vi "Matrix Inverse.vi"(11 "A":sgl[][](array[numeric])) -> (3 "Inverse A":sgl[][](array[numeric]))   [LabVIEW 2017, in "3D Plot.lvclass"]
uses:
  <vilib>/Math Plots/3D Math Plots/3D Plot/3D Plot/3D Plot.lvclass
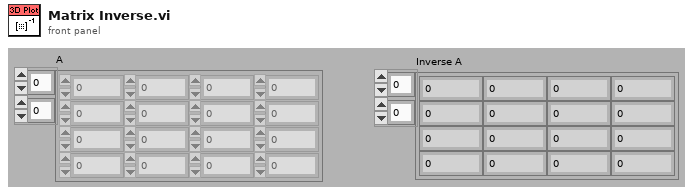
[diagram p1: front panel]
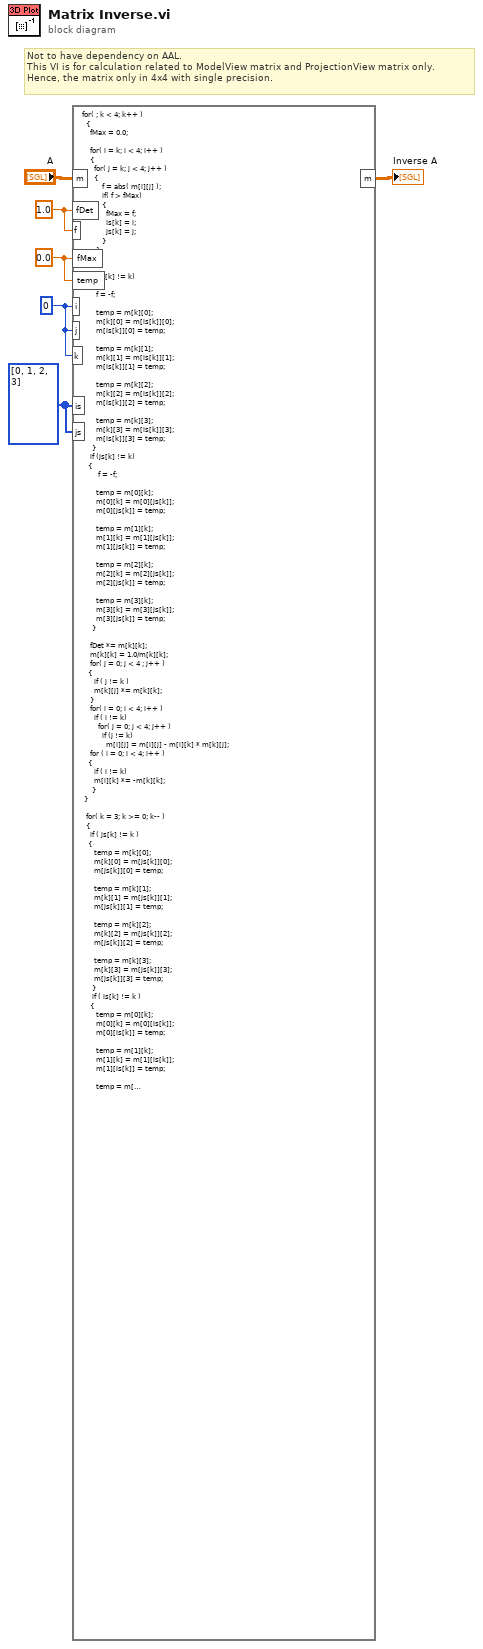
[diagram p0: block diagram]
diagram:
  w3 = 0
  w4 = i32[] [0, 1, 2, 3]
  w5 = sgl 0.0 ("input variable")
  w6 = sgl 1.0 ("input variable")
  # "Not to have dependency on AAL.\nThis VI is for calculation related to ModelView matrix and ProjectionView matrix only.\nHence, the matrix only in 4x4 with single precision."
  n1 = formula code="for( ; k < 4; k++ )\n  {\n    fMax = 0.0;\n\n    for( i = k; i < 4; i++ )\n    {\n      for( j = k; j < 4; j++ )\n      {\n          f = abs( m[i][j] );\n          if( f > fMax)\n          {\n            fMax = f;\n            is[k] = i;\n            js[k] = j;\n          }\n       }\n    }\n  \n    if (is[k] != k)\n  \t{\n       f = -f;\n\n   \t   temp = m[k][0];\n       m[k][0] = m[is[k]][0];\n       m[is[k]][0] = temp;\n\n   \t   temp = m[k][1];\n       m[k][1] = m[is[k]][1];\n       m[is[k]][1] = temp;\n\n   \t   temp = m[k][2];\n       m[k][2] = m[is[k]][2];\n       m[is[k]][2] = temp;\n\n\t      temp = m[k][3];\n       m[k][3] = m[is[k]][3];\n       m[is[k]][3] = temp; \n     }   \n    if (js[k] != k)\n  \t{\n        f = -f;\n  \n\t      temp = m[0][k];\n       m[0][k] = m[0][js[k]];\n       m[0][js[k]] = temp;\n\n\t      temp = m[1][k];\n       m[1][k] = m[1][js[k]];\n       m[1][js[k]] = temp;\n\n\t      temp = m[2][k];\n       m[2][k] = m[2][js[k]];\n       m[2][js[k]] = temp;\n\n\t      temp = m[3][k];\n       m[3][k] = m[3][js[k]];\n       m[3][js[k]] = temp;\n     }\n\n    fDet *= m[k][k];\n    m[k][k] = 1.0/m[k][k];\n    for( j = 0; j < 4 ; j++ )\n   {\n      if ( j != k )\n      m[k][j] *= m[k][k];\n    }\n    for( i = 0; i < 4; i++ )\n      if ( i != k)\n        for( j = 0; j < 4; j++ )\n          if (j != k)\n            m[i][j] = m[i][j] - m[i][k] * m[k][j];\n    for ( i = 0; i < 4; i++ )\n  \t{\n      if ( i != k)\n      m[i][k] *= -m[k][k];\n     }\n }\n\n  for( k = 3; k >= 0; k-- )\n  {\n    if ( js[k] != k )\n  \t{\n\t     temp = m[k][0];\n      m[k][0] = m[js[k]][0];\n      m[js[k]][0] = temp;\n\t  \n   \t  temp = m[k][1];\n      m[k][1] = m[js[k]][1];\n      m[js[k]][1] = temp;\n\n\t     temp = m[k][2];\n      m[k][2] = m[js[k]][2];\n      m[js[k]][2] = temp;\n\n   \t  temp = m[k][3];\n      m[k][3] = m[js[k]][3];\n      m[js[k]][3] = temp;\n     }   \n     if ( is[k] != k )\n    {\n\t      temp = m[0][k];\n       m[0][k] = m[0][is[k]];\n       m[0][is[k]] = temp;\n\n\t      temp = m[1][k];\n       m[1][k] = m[1][is[k]];\n       m[1][is[k]] = temp;\n\n   \t   temp = m[2][k];\n       m[2][k] = m[2][is[k]];\n       m[2][is[k]] = temp;\n\n\t      temp = m[3][k];\n       m[3][k] = m[3][is[k]];\n       m[3][is[k]] = temp;\n      }\n  }"("m"="A", "fDet"=w6, "f"=w6, "fMax"=w5, "temp"=w5, "is"=w4, "js"=w4, "i"=w3, "j"=w3, "k"=w3) -> ("m"=→"Inverse A":sgl[][])
